vi "SubVI_Read_Write_Impedances.vi"(8 "error in (no error)":errorcluster, 11 "LINX Resource in":T1) -> (0 "error out":errorcluster, 2 "LINX Resource out":T1, 3 "Raw Impedances Out":T7)   [LabVIEW 2020]
uses:
  <vilib>/MakerHub/LINX/Private/Type Defs/LINX Ref.ctl
  <vilib>/MakerHub/LINX/Private/Type Defs/Platform.ctl
  <vilib>/MakerHub/LINX/Private/Type Defs/Interface.ctl
  <vilib>/MakerHub/LINX/Private/Device/Type Defs/LINX Device Config.ctl
  <vilib>/MakerHub/LINX/Private/Device/Type Defs/TCP Config.ctl
  <vilib>/MakerHub/LINX/Private/Device/Type Defs/Channels.ctl
  <extravilib>/ChannelInstances/Lossy Stream-a[.](u8)/)Channel.ctl
  <vilib>/MakerHub/LINX/Private/Type Defs/Peripherals/SPI/SPI Configuration.ctl
  <vilib>/MakerHub/LINX/Private/Type Defs/Peripherals/SPI/SPI Bit Order.ctl
  <vilib>/MakerHub/LINX/Private/Type Defs/Peripherals/SPI/SPI Mode.ctl
  <vilib>/MakerHub/LINX/Public/Peripherals/SPI/SPI CS Config.ctl
  <vilib>/MakerHub/LINX/Private/Type Defs/Peripherals/SPI/SPI CS Logic Level.ctl
  <vilib>/MakerHub/LINX/Public/Peripherals/SPI/SPI Write Read 1 Frame.vi
  <vilib>/MakerHub/LINX/Public/Peripherals/SPI/SPI Write Read N Frames.vi
  <extravilib>/ChannelInstances/Lossy Stream-a[.](u8)/Endpoint.vi
  <vilib>/MakerHub/LINX/Private/Local IO/LinxSpiWriteRead.vi
  <vilib>/MakerHub/LINX/Public/Utilities/Check Channel.vi
  <vilib>/MakerHub/LINX/Private/Local IO/Handle Errors.vi
  Global 1.vi
  <vilib>/MakerHub/LINX/Private/Utilties/Generate Error.vi
  <extravilib>/ChannelInstances/Lossy Stream-a[.](u8)/)Channel.vi
  <vilib>/MakerHub/LINX/LMH-LINX.lvlib
  <extravilib>/ChannelInstances/Lossy Stream-a[.](u8).lvlib
  <vilib>/MakerHub/LINX/Private/Device/Device.lvlib
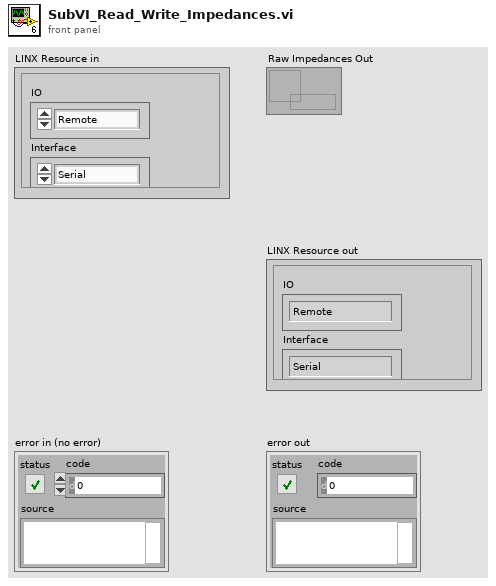
[diagram p1: front panel]
types:
  T1 = typedef "LMH-LINX.lvlib/LINX Ref.ctl" = cluster{"IO":T2, "Interface":T3, "LINX Device Config":T4}
  T2 = typedef "LMH-LINX.lvlib/Platform.ctl" = enum16{"Remote", "Local"}
  T3 = typedef "LMH-LINX.lvlib/Interface.ctl" = enum16{"Serial", "TCP"}
  T4 = typedef "LMH-LINX.lvlib/Device.lvlib/LINX Device Config.ctl" = cluster{"Interface":T3, "COM Port":refnum<visa-resource-name>, "TCP Configuration":T5, "Device Family":u8, "Device ID":u8, "Device Name":string, "TCP Ref":refnum<k5>, "Channels":T6}
  T5 = typedef "LMH-LINX.lvlib/Device.lvlib/TCP Config.ctl" = cluster{"IP Address":string, "Port":u16}
  T6 = typedef "LMH-LINX.lvlib/Channels.ctl" = cluster{"DI":u8[], "DO":u8[], "AI":u8[], "AO":u8[], "PWM":u8[], "QE":u8[], "UART":u8[], "I2C 2":u8[], "SPI":u8[], "CAN":u8[], "Servo":u8[], "AI Ref (V)":dbl, "AI Resolution (Bits)":u8, "AO Ref (V)":dbl, "AO Resolution (Bits)":u8}
  T7 = typedef "Lossy Stream-a[.](u8).lvlib/)Channel.ctl" = refnum<queue>
  T8 = typedef "LMH-LINX.lvlib/SPI CS Config.ctl" = cluster{"CS Channel":u8, "CS Logic Level":T9}
  T9 = typedef "LMH-LINX.lvlib/SPI CS Logic Level.ctl" = enum8{"Active Low", "Active High"}
  T10 = typedef "LMH-LINX.lvlib/SPI Configuration.ctl" = cluster{"Clock Frequency":u32, "Bit Order":T11, "SPI Mode":T12}
  T11 = typedef "LMH-LINX.lvlib/SPI Bit Order.ctl" = enum8{"LSb First", "MSb First"}
  T12 = typedef "LMH-LINX.lvlib/SPI Mode.ctl" = enum8{"Mode 0", "Mode 1", "Mode 2", "Mode 3"}
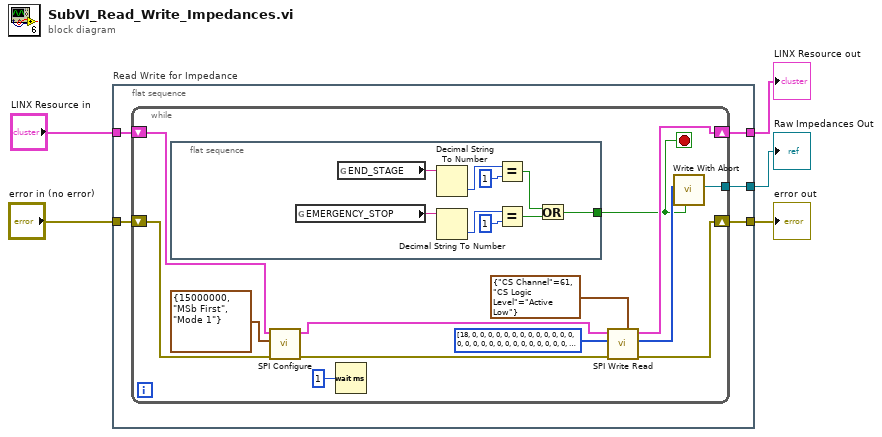
[diagram p0: block diagram]
diagram:
  n1 = flat-sequence "Read Write for Impedance" {
    tunnel: [w10] -> w1
    tunnel: [w9] -> w2
    tunnel: [w8] -> w3
    tunnel: "error in (no error)" -> [w7]
    tunnel: "LINX Resource in" -> [w6]
    frame #0 {
      n2 = while {
        shift-right: [w22] -> w9
        shift-left: w7 -> [w21]
        shift-right: [w20] -> w10
        shift-left: w6 -> [w23]
        tunnel: [w19] -> w8
        stop <- w11 stop-if-true
        n3 = flat-sequence {
          tunnel: [w24] -> w11
          frame #0 {
            n4 = global read "Global 1.vi" "EMERGENCY_STOP"() -> (w27:string)
            n5 = global read "Global 1.vi" "END_STAGE"() -> (w32:string)
            n6 = Decimal String To Number(string=w32) -> (number=w31:i32)  [unwired: 2 in, 1 out]
            n7 = Decimal String To Number(string=w27) -> (number=w29:i32)  [unwired: 2 in, 1 out]
            n8 = Equal?(x=w31, y=1) -> (x = y?=w25:bool)
            n9 = Equal?(x=w29, y=1) -> (x = y?=w26:bool)
            n10 = Or(x=w25, y=w26) -> (x .or. y?=w24:bool)
          }
        }
        n11 = call <vilib>:"SPI Configure.vi"("Error In"=w21, "SPI Configuration"=T10 {"Clock Frequency"=15000000, "Bit Order"=enum."MSb First", "SPI Mode"=enum."Mode 1"}, "LINX Resource"=w23) -> ("Error Out"=w14:errorcluster, "LINX Resource"=w13:T1)  [unwired: 6 in, 1 out]
        n12 = Wait (ms)(milliseconds to wait=u32 1) -> ()  [unwired: 1 out]
        n13 = call-poly <vilib>:"SPI Write Read.vi"("CS Configuration"=T8 {"CS Channel"=61, "CS Logic Level"=enum."Active Low"}, "Error In"=w14, "Data"=u8[] [18, 0, 0, 0, 0, 0, 0, 0, 0, 0, 0, 0, 0, 0, 0, 0, 0, 0, 0, 0, 0, 0, 0, 0, 0, 0, 0, 0, 0, 0, 0], "LINX Resource"=w13) -> ("Error Out"=w22:errorcluster, "Read Data"=w15:u8[], "LINX Resource"=w20:T1)  [unwired: 4 in, 1 out]
        n14 = call <extravilib>:"Write With Abort.vi"("abort"=w11, "element"=w15) -> ("channel"=w19:T7)  [unwired: 6 in, 3 out]
      }
    }
  }
  "Raw Impedances Out" <- w3
  "error out" <- w2
  "LINX Resource out" <- w1
